vi "voltaje.vi"(7 "VISA resource name":refnum<visa-resource-name>, 8 "Unit(V)":u16(ring) items=["V", "mV", "kV", "A", "mA"], 9 "Function(0:Voltage)":u16(ring) items=["Voltage", "Current"], 10 "Measurement Function (0:Voltage)":u16(ring) items=["Voltage", "Current", "Power"], 11 "Valor del voltaje":dbl) -> (1 "Valor voltaje":dbl, 2 "corriente":dbl)   [LabVIEW 2016]
doc: "En este subVI se controla la fuente de voltaje por medio de los subVIs que proporciona el fabricante de la fuente.\n\nComo entradas tiene el tipo de medición que se quiere realizar, las unidades entre otros, además del valor de voltaje que se desea aplicar a la muestra. \n\nComo salidas están los valores de voltaje y corriebnte que propociona la fuente."
uses:
  <instrlib>/Keithley 2200 Series/Keithley 2200 Series.lvlib
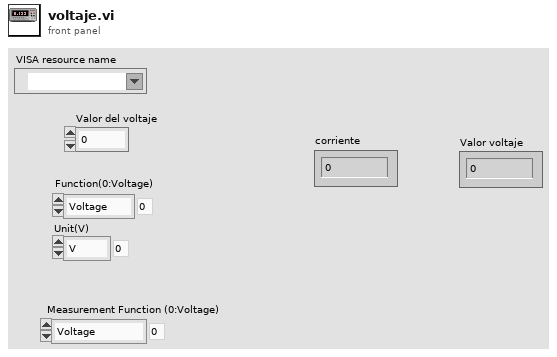
[diagram p1: front panel]
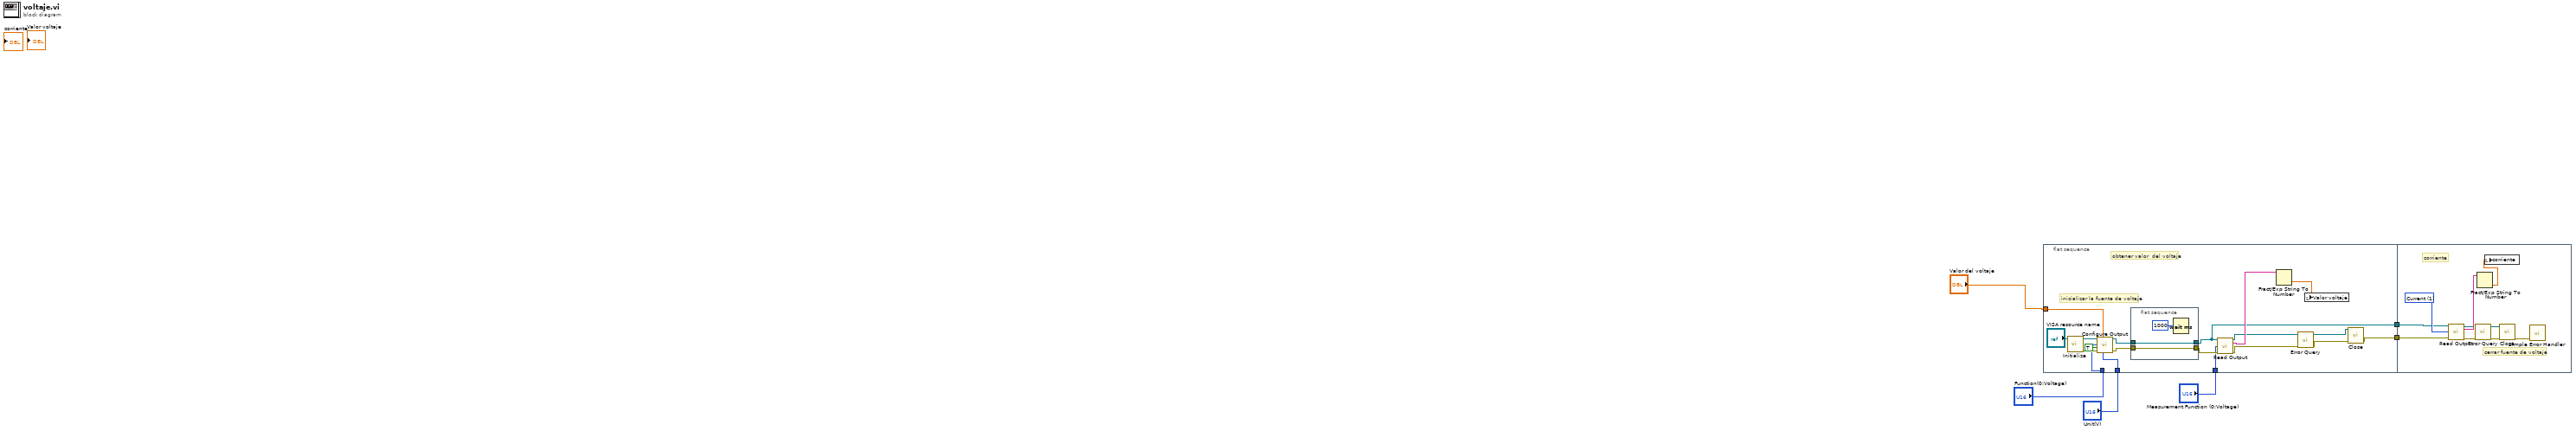
[diagram p0: block diagram]
diagram:
  n1 = flat-sequence {
    tunnel: "Valor del voltaje" -> [w18]
    tunnel: "Function(0:Voltage)" -> [w10]
    tunnel: "Measurement Function (0:Voltage)" -> [w17]
    tunnel: [w12] -> w6
    tunnel: [w11] -> w5
    tunnel: "Unit(V)" -> [w8]
    tunnel: w6 -> [w33]
    tunnel: w5 -> [w38]
    frame #0 {
      # "inicializar la fuente de voltaje"
      # "obtener valor  del voltaje"
      n2 = call <instrlib>:"Initialize.vi"("VISA resource name"="VISA resource name") -> ("error out"=w24:errorcluster, "VISA resource name out"=w25:refnum<visa-resource-name>)  [unwired: 9 in]
      n3 = call <instrlib>:"Configure Output.vi"("VISA resource name"=w25, "Manual Range(0.00)"=w18, "Function(0:Voltage)"=w10, "Enable Output (T: Enable)"=TRUE, "error in (no error)"=w24, "Unit(V)"=w8) -> ("VISA resource name out"=w22:refnum<visa-resource-name>, "error out"=w21:errorcluster)  [unwired: 8 in]
      n4 = flat-sequence {
        tunnel: w21 -> [w27]
        tunnel: [w27] -> w20
        tunnel: w22 -> [w26]
        tunnel: [w26] -> w12
        frame #0 {
          n5 = Wait (ms)(milliseconds to wait=u32 1000) -> ()  [unwired: 1 out]
        }
      }
      n6 = call <instrlib>:"Read Output.vi"("VISA resource name"=w12, "Measurement Function (0:Voltage)"=w17, "error in (no error)"=w20) -> ("VISA resource name out"=w16:refnum<visa-resource-name>, "Measurement"=w19:string, "error out"=w15:errorcluster)  [unwired: 10 in]
      n7 = Fract/Exp String To Number(string=w19) -> (number=w9:dbl)  [unwired: 3 in, 1 out]
      n8 = call <instrlib>:"Error Query.vi"("error in (no error)"=w15, "VISA resource name"=w16) -> ("error out"=w14:errorcluster, "VISA resource name out"=w13:refnum<visa-resource-name>)  [unwired: 6 in, 2 out]
      n9 = local write "Valor voltaje"(w9) -> ()
      n10 = call <instrlib>:"Close.vi"("error in (no error)"=w14, "VISA resource name"=w13) -> ("error out"=w11:errorcluster)  [unwired: 9 in]
    }
    frame #1 {
      w37 = u16 1 items=["Voltage", "Current", "Power"] ("Measurement Function (0:Voltage)")
      # "cerrar fuente de voltaje"
      # "corriente"
      n11 = call <instrlib>:"Read Output.vi"("VISA resource name"=w33, "Measurement Function (0:Voltage)"=w37, "error in (no error)"=w38) -> ("VISA resource name out"=w35:refnum<visa-resource-name>, "Measurement"=w36:string, "error out"=w34:errorcluster)  [unwired: 10 in]
      n12 = call <instrlib>:"Error Query.vi"("error in (no error)"=w34, "VISA resource name"=w35) -> ("error out"=w29:errorcluster, "VISA resource name out"=w30:refnum<visa-resource-name>)  [unwired: 6 in, 2 out]
      n13 = Fract/Exp String To Number(string=w36) -> (number=w32:dbl)  [unwired: 3 in, 1 out]
      n14 = local write "corriente"(w32) -> ()
      n15 = call <instrlib>:"Close.vi"("error in (no error)"=w29, "VISA resource name"=w30) -> ("error out"=w31:errorcluster)  [unwired: 9 in]
      n16 = call <vilib>:"Simple Error Handler.vi"("error in (no error)"=w31) -> ()  [unwired: 4 in, 5 out]
    }
  }
